vi "Receive Panel Close Event.vi"(8 "error in (no error)":errorcluster, 10 "PanelCloseMsg":refnum<class "PanelCloseMsg.lvclass">, 11 "IViewModel In":refnum<class "IViewModel.lvclass">) -> (0 "error out":errorcluster, 3 "IViewModel Out":refnum<class "IViewModel.lvclass">)   [LabVIEW 2018, in "MVA Framework.lvlib" / "IViewModel.lvlib" / "IViewModel.lvclass"]
doc: "接收面板关闭事件"
uses:
  IViewModel.lvclass
  <vilib>/ActorFramework/Actor/Actor.lvclass
  <vilib>/ActorFramework/Stop Msg/Stop Msg.lvclass
  ActorEvents/IEventAggregator Messages/PanelCloseMsg/PanelCloseMsg.lvclass
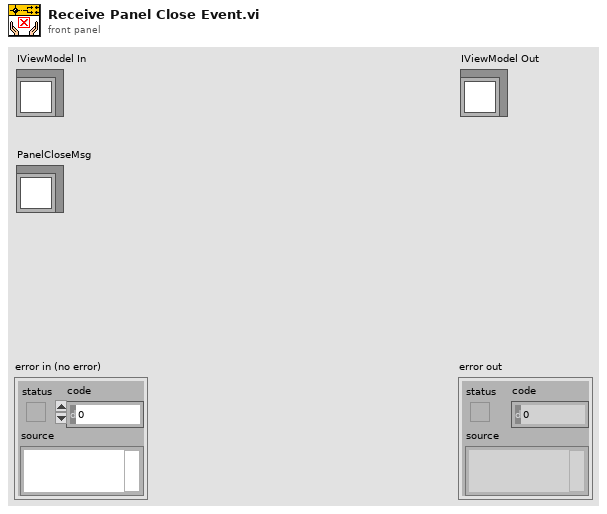
[diagram p1: front panel]
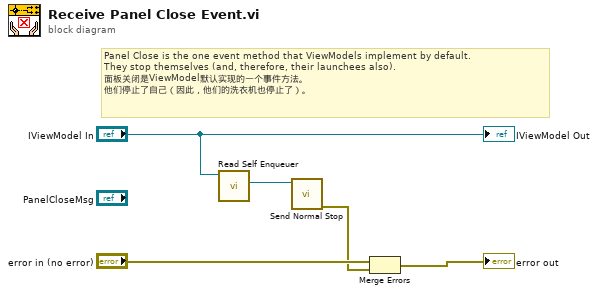
[diagram p0: block diagram]
diagram:
  # "Panel Close is the one event method that ViewModels implement by default.\nThey stop themselves (and, therefore, their launchees also).\n面板关闭是ViewModel默认实现的一个事件方法。\n他们停止了自己（因此，他们的洗衣机也停止了）。"
  n1 = call <vilib>:"Read Self Enqueuer.vi"("Actor"="IViewModel In") -> ("Self Enqueuer"=w4:refnum<class "Message Enqueuer.lvclass">)  [unwired: 10 in]
  n2 = call <vilib>:"Send Normal Stop.vi"("Message Enqueuer"=w4) -> ("error out"=w2:errorcluster)  [unwired: 10 in]
  n3 = Merge Errors("error in (no error)", w2) -> (→"error out":errorcluster)
  "IViewModel Out" <- "IViewModel In"
